vi "Get Buffer.vi"(11 "Thermometer DAQmx RTD Cont CFG in":refnum<class "Thermometer DAQmx RTD Cont CFG.lvclass">) -> (2 "Buffer Lossless DBL":refnum<class "Buffer Lossless DBL.lvclass">, 3 "Thermometer DAQmx RTD Cont CFG out":refnum<class "Thermometer DAQmx RTD Cont CFG.lvclass">)   [LabVIEW 2024, in "Thermometer DAQmx RTD Cont CFG.lvclass"]
uses:
  Thermometer DAQmx RTD Cont CFG.lvclass
  Thermometer DAQmx RTD Cont CFG.lvclass/Thermometer DAQmx RTD Cont CFG.ctl
  Buffers/Buffer Lossless DBL/Buffer Lossless DBL.lvclass
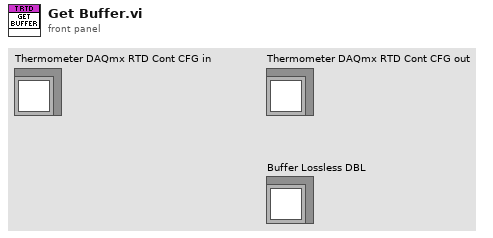
[diagram p1: front panel]
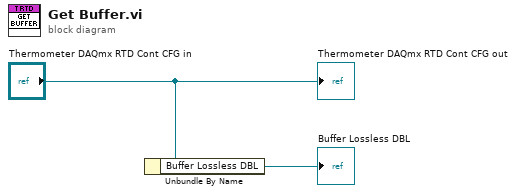
[diagram p0: block diagram]
diagram:
  n1 = Unbundle By Name("Thermometer DAQmx RTD Cont CFG in") -> ("Buffer Lossless DBL"=→"Buffer Lossless DBL":refnum<class "Buffer Lossless DBL.lvclass">)
  "Thermometer DAQmx RTD Cont CFG out" <- "Thermometer DAQmx RTD Cont CFG in"
